vi "JSON GRUPO 3.vi"(8 "error in":errorcluster, 11 "Result":T1(array[cluster])) -> (0 "error IO":errorcluster, 3 "Generador":refnum<class "JSON Object.lvclass">[](array[class]))   [LabVIEW 2015]
uses:
  <vilib>/addons/JSON API/Get Polymorphic/JSON GetSet.lvlib
  <vilib>/addons/JSON API/JSON Object/Set Object Item by name.vi
  <vilib>/addons/JSON API/JSON Object/JSON Object.lvclass
  <vilib>/addons/JSON API/JSON Array/Set JSON Array.vi
  <vilib>/addons/JSON API/JSON Array/JSON Array.lvclass
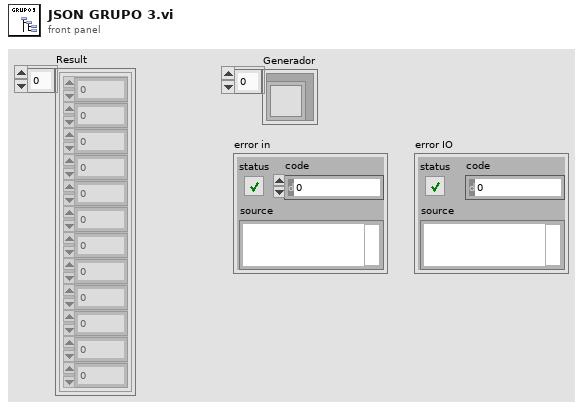
[diagram p1: front panel]
types:
  T1 = cluster{u32, dbl, dbl, dbl, dbl, dbl, dbl, dbl, dbl, dbl, dbl, dbl}[]
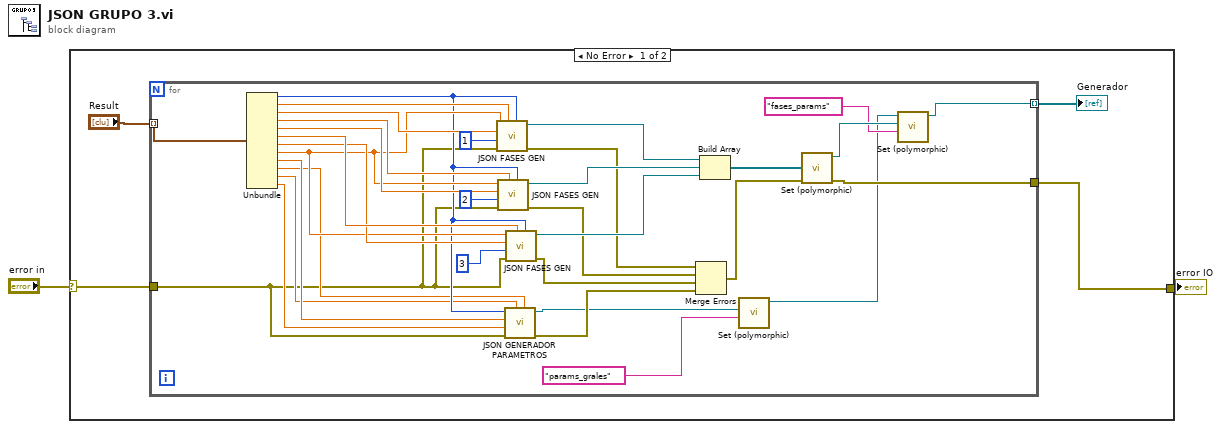
[diagram p0: block diagram]
diagram:
  n1 = case shown="No Error" "error in" {
    selector: "error in" -> [w5 w40]
    tunnel: [w6 w40] -> w2
    frame No Error {
      n2 = for {
        tunnel: "Result" -> [w39] mode=indexing
        tunnel: w5 -> [w13]
        tunnel: [w20] -> w6
        tunnel: [w8] -> w3 mode=indexing
        n3 = Unbundle(w39) -> (w19:u32, w38:dbl, w37:dbl, w35:dbl, w34:dbl, w32:dbl, w31:dbl, w30:dbl, w18:dbl, w17:dbl, w16:dbl, w15:dbl)
        n4 = call "JSON FASES GEN.vi"("time"=w19, "Tension"=w38, "error in"=w13, "Fase"=u32 1, "Corriente"=w37, "Potencia"=w30) -> ("error out"=w25:errorcluster, "JSON Object out"=w28:refnum<class "JSON Object.lvclass">)  [unwired: 4 in]
        n5 = call "JSON FASES GEN.vi"("time"=w19, "Tension"=w35, "error in"=w13, "Fase"=u32 2, "Corriente"=w34, "Potencia"=w30) -> ("error out"=w24:errorcluster, "JSON Object out"=w27:refnum<class "JSON Object.lvclass">)  [unwired: 4 in]
        n6 = call "JSON GENERADOR PARAMETROS.vi"("enige_hours"=w17, "power_gen"=w16, "error in"=w13, "power_factor"=w15, "fuel_usage"=w18, "time"=w19) -> ("error out"=w14:errorcluster, "JSON Object out"=w12:refnum<class "JSON Object.lvclass">)  [unwired: 4 in]
        n7 = call "JSON FASES GEN.vi"("time"=w19, "Tension"=w32, "error in"=w13, "Fase"=u32 3, "Corriente"=w31, "Potencia"=w30) -> ("error out"=w23:errorcluster, "JSON Object out"=w26:refnum<class "JSON Object.lvclass">)  [unwired: 4 in]
        n8 = Merge Errors(w25, w24, w23, w14) -> (w21:errorcluster)
        n9 = Build Array(w28, w27, w26) -> (w22:refnum<class "JSON Object.lvclass">[])
        n10 = call-poly <vilib>:"Set (polymorphic).vi"("name"="params_grales", "Value"=w12) -> ("JSON Object out"=w7:refnum<class "JSON Object.lvclass">)  [unwired: 7 in, 2 out]
        n11 = call-poly <vilib>:"Set (polymorphic).vi"("error in (no error)"=w21, "Array"=w22) -> ("error out"=w20:errorcluster, "JSON Array out"=w10:refnum<class "JSON Array.lvclass">)  [unwired: 8 in]
        n12 = call-poly <vilib>:"Set (polymorphic).vi"("name"="fases_params", "Value"=w10, "JSON Object in"=w7) -> ("JSON Object out"=w8:refnum<class "JSON Object.lvclass">)  [unwired: 6 in, 2 out]
      }
      "Generador" <- w3
    }
    frame Error {
    }
  }
  "error IO" <- w2
